vi "Send Status String to UI.vi"(8 "error in (no error)":errorcluster, 10 "Status String to Send":string, 11 "object in":refnum<class "_test class base.lvclass">) -> (0 "error out":errorcluster, 3 "object out":refnum<class "_test class base.lvclass">)   [LabVIEW 2013, in "_test class base.lvlib" / "_test class base.lvclass"]
uses:
  _test class base.lvclass
  <vilib>/ActorFramework/Actor/Actor.lvclass/Actor.ctl
  Tesla Factory Tester/Messages/Update Status String_Msg/Update Status String_Msg.lvclass/Update Status String_Msg.ctl
  <vilib>/ActorFramework/Message Enqueuer/Message Enqueuer.lvclass/Message Enqueuer.ctl
  <vilib>/ActorFramework/Message Enqueuer/Enqueue.vi
  <vilib>/ActorFramework/Message Priority Queue/Priority Enqueue.vi
  Tesla Factory Tester/Messages/Update Status String_Msg/Update Status String_Msg.lvclass
  <vilib>/ActorFramework/Actor/Actor.lvclass
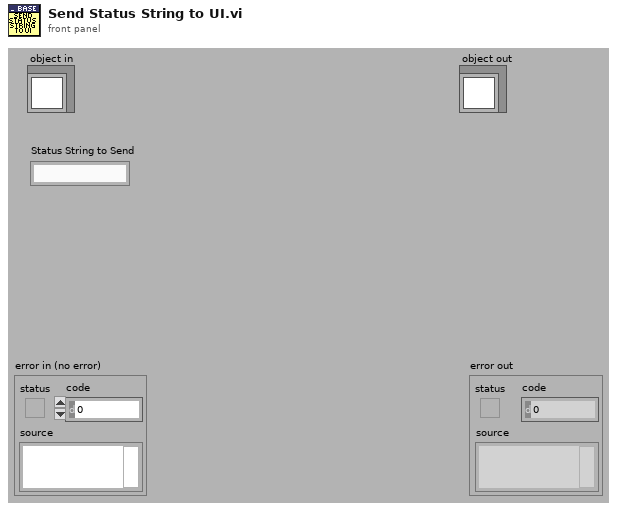
[diagram p1: front panel]
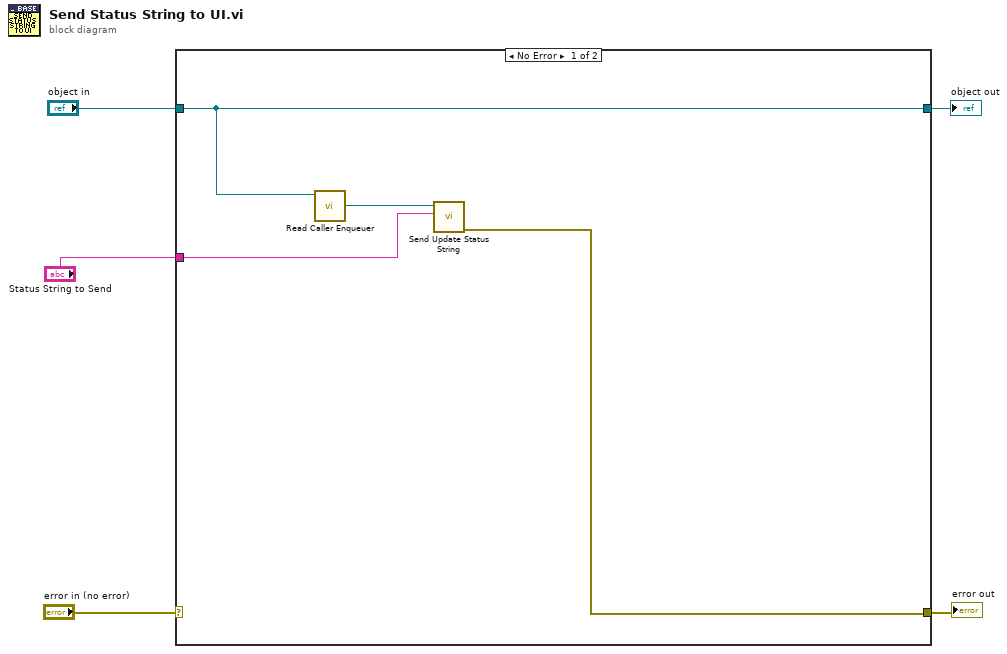
[diagram p0: block diagram]
diagram:
  n1 = case shown="No Error" "error in (no error)" {
    selector: "error in (no error)" -> [_ w11]
    tunnel: [w6 w11] -> w4
    tunnel: [w9 w10] -> w2
    tunnel: "object in" -> [w9 w10]
    tunnel: "Status String to Send" -> [w7 _]
    frame No Error {
      n2 = call <vilib>:"Read Caller Enqueuer.vi"("Actor"=w9) -> ("Caller Enqueuer"=w8:refnum<class "Message Enqueuer.lvclass">)  [unwired: 10 in]
      n3 = call "Send Update Status String.vi"("Append this string"=w7, "Message Enqueuer"=w8) -> ("error out"=w6:errorcluster)  [unwired: 8 in, 1 out]
    }
    frame Error {
    }
  }
  "error out" <- w4
  "object out" <- w2
